vi "climb teleop.vi"(9 "POV":i16) -> ()   [LabVIEW 2019]
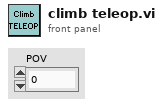
[diagram p1: front panel]
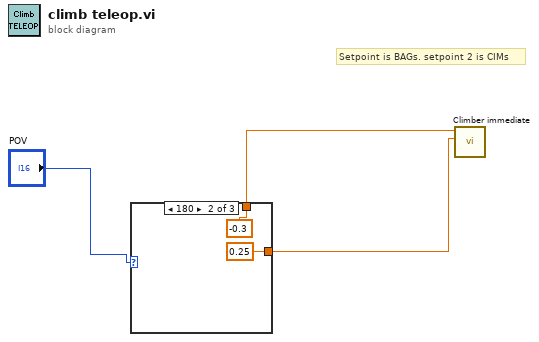
[diagram p0: block diagram]
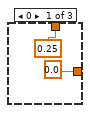
[diagram p2: hidden frame]
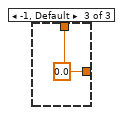
[diagram p3: hidden frame]
diagram:
  # "Setpoint is BAGs. setpoint 2 is CIMs"
  n1 = case shown="180" "POV" {
    tunnel: [0.0 0.25 w8] -> w2
    tunnel: [0.25 -0.3 w8] -> w1
    frame 0 {
    }
    frame 180 {
    }
    frame -1, Default {
      w8 = 0.0
    }
  }
  n2 = call "Climber immediate.vi"("Lift"=w2, "Elevation"=w1) -> ()  [unwired: 9 in, 1 out]
